vi "Periodic Tasks.vi"(8 "error in":errorcluster) -> ()   [LabVIEW 2023]
doc: "This VI runs in parallel to other tasks. It can contain as many user-defined periodic loops as you need. These can carry out PID or other sorts of timed response."
uses:
  <vilib>/Rock Robotics/WPI/DriverStation/WPI_DriverStationAllianceInfo.ctl
  <vilib>/Rock Robotics/Network Tables/NT Read String.vi
  <vilib>/Rock Robotics/Network Tables/NT Write String.vi
  GeneralPurpose/AllianceColorGlobal.vi
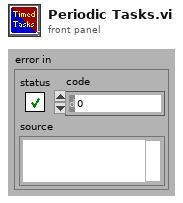
[diagram p1: front panel]
types:
  T1 = typedef "WPI_DriverStationAllianceInfo.ctl" = enum16{"Red", "Blue", "Invalid"}
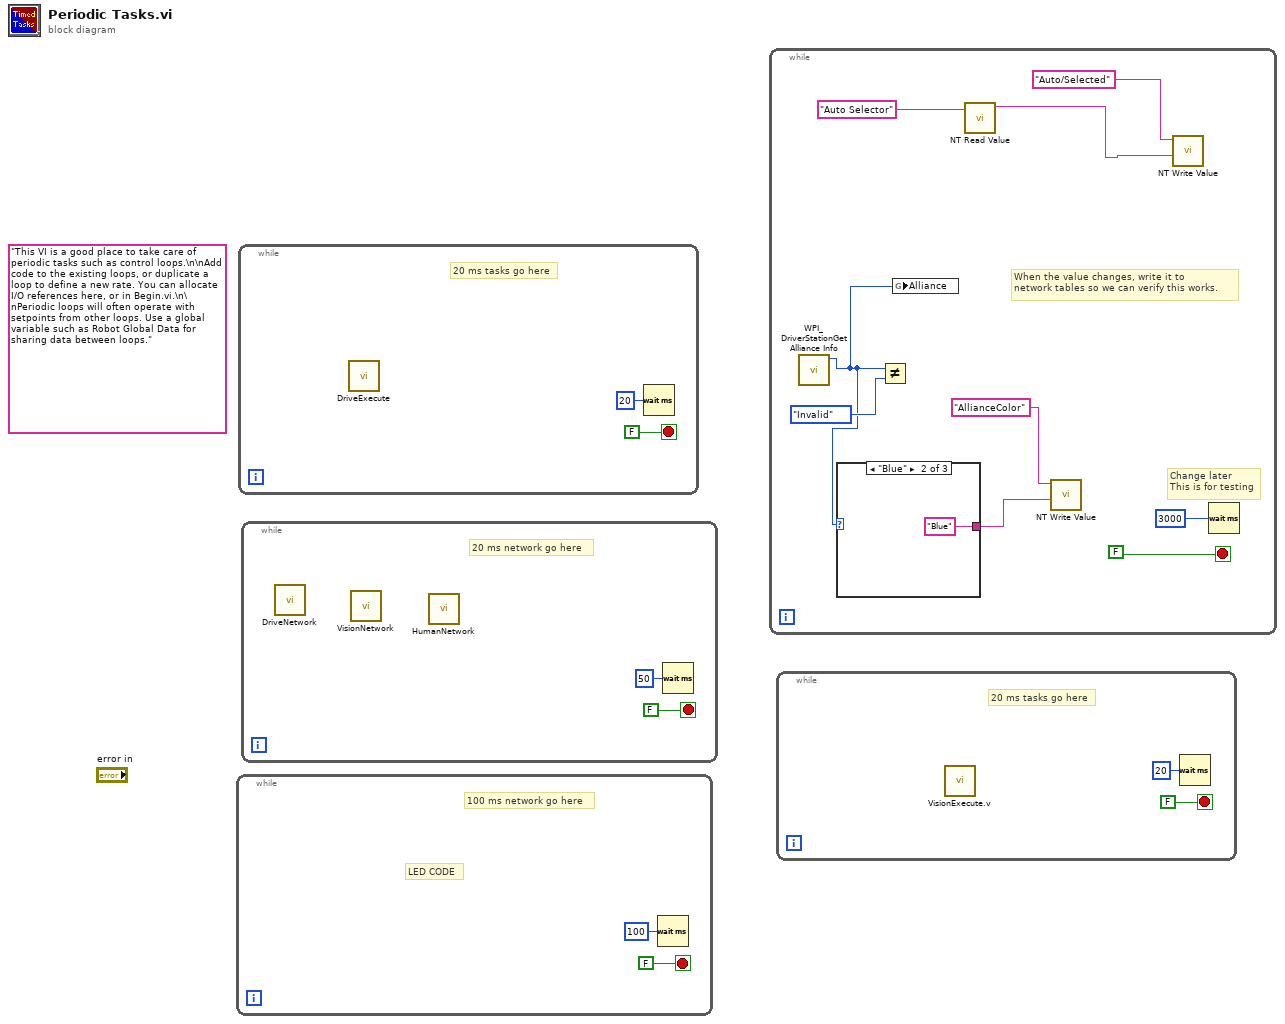
[diagram p0: block diagram]
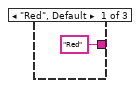
[diagram p2: hidden frame]
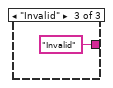
[diagram p3: hidden frame]
diagram:
  (unwired) "This VI is a good place to take care of periodic tasks such as control loops.\n\nAdd code to the existing loops, or duplicate a loop to define a new rate. You can allocate I/O references here, or in Begin.vi.\n\nPeriodic loops will often operate with setpoints from other loops. Use a global variable such as Robot Global Data for sharing data between loops."
  n1 = while {
    stop <- FALSE stop-if-true
    # "LED CODE"
    # "100 ms network go here"
    n2 = Wait (ms)(milliseconds to wait=u32 100) -> ()  [unwired: 1 out]
  }
  n3 = while {
    stop <- FALSE stop-if-true
    # "20 ms tasks go here"
    n4 = call "DriveExecute.vi"() -> ()  [unwired: 11 in, 1 out]
    n5 = Wait (ms)(milliseconds to wait=u32 20) -> ()  [unwired: 1 out]
  }
  n6 = while {
    stop <- FALSE stop-if-true
    # "20 ms network go here"
    n7 = call "DriveNetwork.vi"() -> ()  [unwired: 11 in, 1 out]
    n8 = call "VisionNetwork.vi"() -> ()  [unwired: 11 in, 1 out]
    n9 = call "HumanNetwork.vi"() -> ()  [unwired: 11 in, 1 out]
    n10 = Wait (ms)(milliseconds to wait=u32 50) -> ()  [unwired: 1 out]
  }
  n11 = while {
    stop <- FALSE stop-if-true
    # "When the value changes, write it to \nnetwork tables so we can verify this works."
    # "Change later\nThis is for testing"
    n12 = call <vilib>:"WPI_DriverStationGet Alliance Info.vi"() -> ("Alliance"=w12:T1)  [unwired: 6 in, 5 out]
    n13 = case shown="\"Blue\"" w12 {
      tunnel: ["Red" "Blue" "Invalid"] -> w11
      frame "Red", Default {
      }
      frame "Blue" {
      }
      frame "Invalid" {
      }
    }
    n14 = Not Equal?(x=w12, y=WPI_DriverStationAllianceInfo."Invalid") -> ()  [unwired: 1 out]
    n15 = global write "AllianceColorGlobal.vi" "Alliance"(w12) -> ()
    n16 = call-poly <vilib>:"NT Read Value.vi"("name"="Auto Selector" ("Name")) -> ("value"=w7:string)  [unwired: 8 in, 2 out]
    n17 = call-poly <vilib>:"NT Write Value.vi"("value"=w11, "name"="AllianceColor") -> ()  [unwired: 9 in, 1 out]
    n18 = call-poly <vilib>:"NT Write Value.vi"("value"=w7, "name"="Auto/Selected") -> ()  [unwired: 9 in, 1 out]
    n19 = Wait (ms)(milliseconds to wait=u32 3000) -> ()  [unwired: 1 out]
  }
  n20 = while {
    stop <- FALSE stop-if-true
    # "20 ms tasks go here"
    n21 = call "VisionExecute.v.vi"() -> ()  [unwired: 12 in]
    n22 = Wait (ms)(milliseconds to wait=u32 20) -> ()  [unwired: 1 out]
  }
